vi "SoftwareFrequency.vi"() -> ()   [LabVIEW 2012]
panel:
  in  "Signal Frequency":dbl=600.0 caption="Frequency"
  out "Measured Freq":dbl
  in  "stop":bool
  # "This example takes one second of a square signal\nand counts the rising edges in order to determine the frequency of the\nsignal.  In order to do this, the inside loop compares each data point\nto the previous.  If the current data point is larger than previous, there\nmust have been a rising edge and we increment our count.\n\nThis example will only measure frequencies up to 50kHz.  Any larger \nand you must increase the sample rate of the simulated signal and also\nthe number of samples to match."
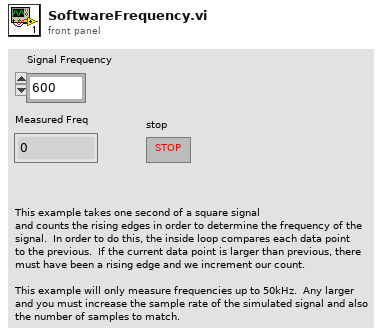
[diagram p1: front panel]
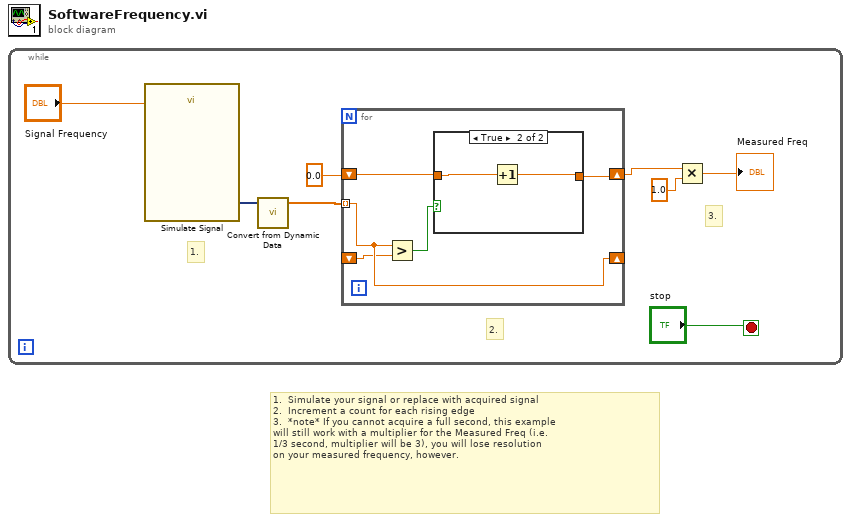
[diagram p0: block diagram]
diagram:
  # "1.  Simulate your signal or replace with acquired signal\n2.  Increment a count for each rising edge\n3.  *note* If you cannot acquire a full second, this example\nwill still work with a multiplier for the Measured Freq (i.e. \n1/3 second, multiplier will be 3), you will lose resolution \non your measured frequency, however."
  n1 = while {
    stop <- "stop" stop-if-true
    # "3."
    # "2."
    # "1."
    n2 = call "Simulate Signal"("Frequency"="Signal Frequency") -> ("Square"=w7:dynamicdata)  [unwired: 13 in, 1 out]
    n3 = call "Convert from Dynamic Data"("Dynamic Data Type"=w7) -> ("Array"=w6:dbl[])  [unwired: 3 in]
    n4 = for {
      tunnel: w6 -> [w13] mode=indexing
      shift-right: [w13] -> _
      shift-left: _ -> [w12]
      shift-right: [w9] -> w3
      shift-left: 0.0 -> [w10]
      n5 = Greater?(x=w13, y=w12) -> (0:w11:bool)
      n6 = case shown="True" w11 {
        tunnel: w10 -> [w14 w16]
        tunnel: [w14 w15] -> w9
        frame False {
        }
        frame True {
          n7 = Increment(x=w16) -> (x+1=w15:dbl)
        }
      }
    }
    n8 = Multiply(x=w3, y=1.0) -> (x*y=→"Measured Freq":dbl)
  }
